vi "Get Desired Size.vi"(8 "error in (no error)":errorcluster, 11 "ExBlank in":refnum<class "ExBlank.lvclass">) -> (0 "error out":errorcluster, 2 "Desired Size":T1, 3 "ExBlank out":refnum<class "ExBlank.lvclass">)   [LabVIEW 2020, in "2D Array Example.lvlib" / "ExBlank.lvclass"]
uses:
  ExBlank.lvclass
  OOPanel/Desired Size.ctl
  OOPanel/OOPanel.lvlib
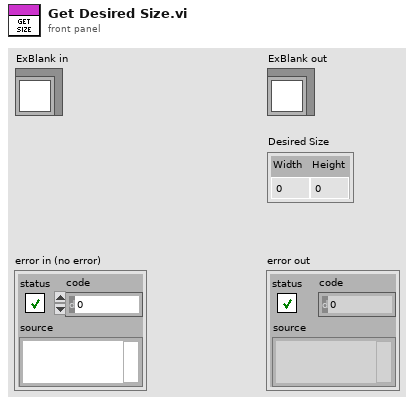
[diagram p1: front panel]
types:
  T1 = typedef "OOPanel.lvlib/Desired Size.ctl" = cluster{"Width":u32, "Height":u32}
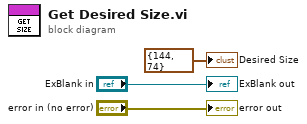
[diagram p0: block diagram]
diagram:
  "error out" <- "error in (no error)"
  "ExBlank out" <- "ExBlank in"
  "Desired Size" <- T1 {"Width"=144, "Height"=74} ("Desired Size")
